vi "dboard eeprom get revision.vi"(8 "error in (no error)":errorcluster, 10 "revision_out":i32, 11 "h":u64) -> (0 "error out":errorcluster, 2 "revision_out out":i32, 3 "function return":u32(ring))   [LabVIEW 2023, in "uhd.lvlib"]
doc: "UHD_API uhd_error uhd_dboard_eeprom_get_revision(\n uhd_dboard_eeprom_handle h, int* revision_out);"
uses:
  <userlib>/uhd/uhd.lvlib
  <userlib>/uhd/uhd.dll
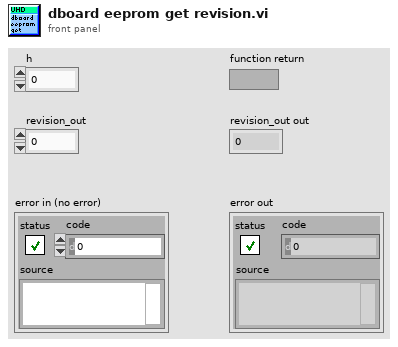
[diagram p1: front panel]
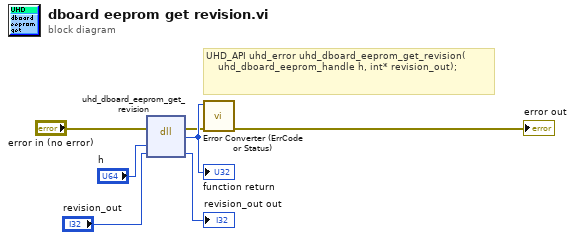
[diagram p0: block diagram]
diagram:
  # "UHD_API uhd_error uhd_dboard_eeprom_get_revision(\n    uhd_dboard_eeprom_handle h, int* revision_out);"
  n1 = dll-call lib="C:/Program Files/National Instruments/LabVIEW 2023/user.lib/uhd/uhd.*" fn="uhd_dboard_eeprom_get_revision"(error in="error in (no error)", "h"="h", "revision_out"="revision_out") -> (error out=w2:errorcluster, w7:u32, "revision_out"=→"revision_out out":i32)  [unwired: 3 in, 1 out]
  "function return" <- w7
  n2 = call <userlib>:"Error Converter (ErrCode or Status).vi"("error in (no error)"=w2, "error code"=w7) -> ("error out"=→"error out":errorcluster)  [unwired: 9 in]
